vi "Uninstall All Software.vi"(6 "Target Config":T1={"IP Address"="0.0.0.0", "Target"=enum."cRIO-9012", "Username"="", "Password"=""}, 8 "error in (no error)":errorcluster, 10 "Sys Cfg Session In":refnum<k21>, 11 "Console Ref In":refnum<vi>) -> (0 "error out":errorcluster, 2 "Sys Cfg Session Out":refnum<k21>, 3 "Console Ref Out":refnum<vi>)   [LabVIEW 2015]
doc: "Uninstall all software from the target."
uses:
  Type Defs/Target Config Cluster.ctl
  Type Defs/RT Target Type.ctl
  <vilib>/nisyscfg/Uninstall All.vi
  <vilib>/nisyscfg/nisyscfg.lvlib
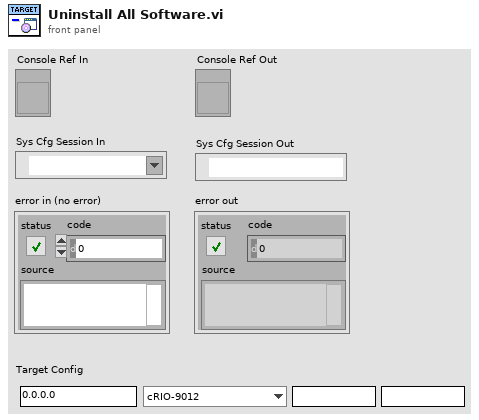
[diagram p1: front panel]
types:
  T1 = typedef "Target Config Cluster.ctl" = cluster{"IP Address":string, "Target":T2, "Username":string, "Password":string}
  T2 = typedef "RT Target Type.ctl" = enum16{"cRIO-9012", "cRIO-9014", "cRIO-9022", "cRIO-9023", "cRIO-9024", "cRIO-9025", "cRIO-9068", "cRIO-9073", "cRIO-9074", "cRIO-9075", "cRIO-9076", "cRIO-9081", "cRIO-9082", "myRIO-1900", "myRIO-1950", "PXI-8101", "PXI-8115", "PXI-8119", "PXI-8820", "PXIe-8100", "PXIe-8101", "PXIe-8133", "PXIe-8135", "PXIe-8820", "sbRIO-9605", "sbRIO-9606", "sbRIO-9623", "sbRIO-9626", "sbRIO-9633", "sbRIO-9636", "Unlisted (Linux-RT)", "Unlisted (PharLap)", "Unlisted (VxWorks)"}
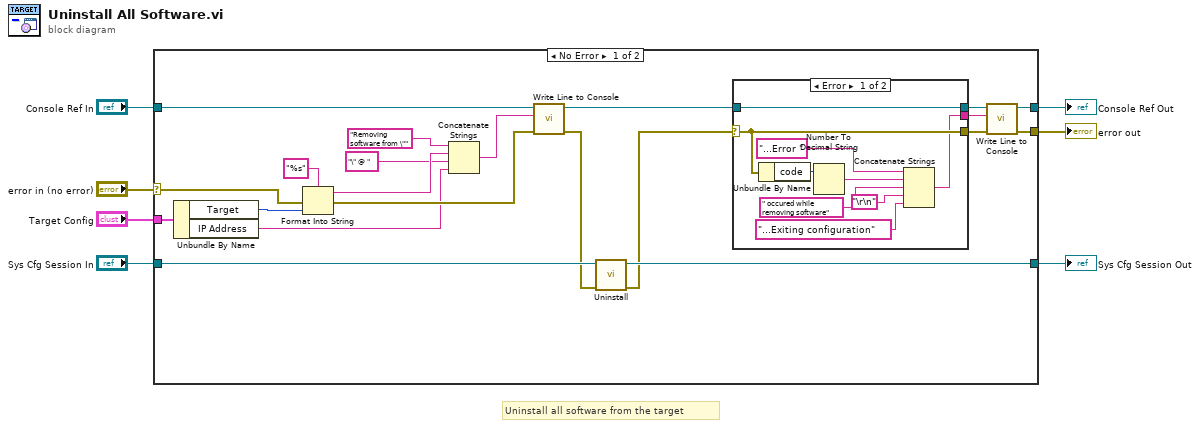
[diagram p0: block diagram]
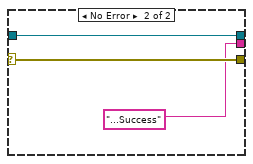
[diagram p2: hidden frame]
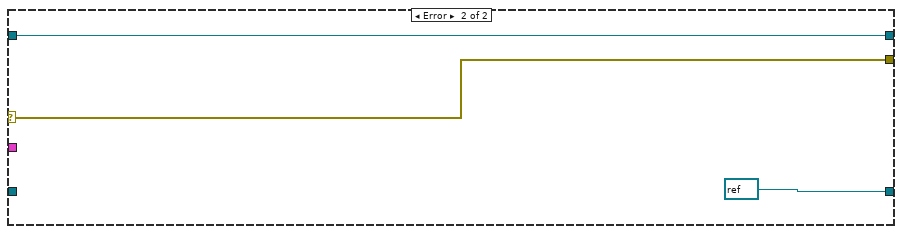
[diagram p3: hidden frame]
diagram:
  # "Uninstall all software from the target"
  n1 = case shown="No Error" "error in (no error)" {
    selector: "error in (no error)" -> [w25 w42]
    tunnel: "Console Ref In" -> [w21 w43]
    tunnel: "Target Config" -> [w28 _]
    tunnel: [w14 w43] -> w4
    tunnel: [w13 w42] -> w3
    tunnel: [w9 refnum<k21> refnum ("session out")] -> w2
    tunnel: "Sys Cfg Session In" -> [w11 _]
    frame No Error {
      n2 = Unbundle By Name(w28) -> ("Target"=w27:T2, "IP Address"=w12:string)
      n3 = Format Into String(format string="%s", error in=w25, w27) -> (resulting string=w23:string, error out=w20:errorcluster)  [unwired: 1 in]
      n4 = Concatenate Strings("Removing software from \"", w23, "\" @ ", w12) -> (w19:string)
      n5 = call "Write Line to Console.vi"("error in (no error)"=w20, "Line to Write"=w19, "Console Ref In"=w21) -> ("error out (no error)"=w10:errorcluster, "Console Ref In Out"=w18:refnum<vi>)  [unwired: 7 in]
      n6 = call-poly <vilib>:"Uninstall.vi"("error in (no error)"=w10, "Session in"=w11) -> ("error out"=w8:errorcluster, "Session out"=w9:refnum<k21>)  [unwired: 8 in]
      n7 = case shown="Error" w8 {
        selector: w8 -> [w36 w39]
        tunnel: w18 -> [w37 w40]
        tunnel: [w37 w40] -> w17
        tunnel: [w36 w39] -> w16
        tunnel: [w29 "...Success"] -> w15
        frame Error {
          n8 = Unbundle By Name(w36) -> ("code"=w35:i32)
          n9 = Number To Decimal String(number=w35) -> (decimal integer string=w34:string)  [unwired: 1 in]
          n10 = Concatenate Strings("...Error ", w34, " occured while removing software", "\r\n", "...Exiting configuration") -> (w29:string)
        }
        frame No Error {
        }
      }
      n11 = call "Write Line to Console.vi"("error in (no error)"=w16, "Line to Write"=w15, "Console Ref In"=w17) -> ("error out (no error)"=w13:errorcluster, "Console Ref In Out"=w14:refnum<vi>)  [unwired: 7 in]
    }
    frame Error {
    }
  }
  "error out" <- w3
  "Console Ref Out" <- w4
  "Sys Cfg Session Out" <- w2
